vi "Wärmepumpe.WriteZustandsgrössen.vi"(0 "Wärmepumpe in":refnum<data-value>, 1 "Vorlauftemperatur \nHeizkreislauf [°C] WPM":dbl, 2 "Vorlauftemperatur \nSolekreislauf [°C] WPM":dbl, 3 "Verdichter 1":bool, 4 "Verdichter 2":bool, 5 "Error in":errorcluster) -> (19 "Error out":errorcluster)   [LabVIEW 2016, in "Wärmepumpe.lvclass"]
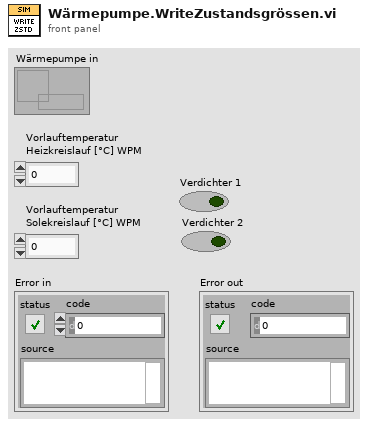
[diagram p1: front panel]
types:
  T1 = typedef "Wärmepumpe.lvclass/Wärmepumpe.Zustandsgrössen.ctl" = cluster{"Vorlauftemperatur Heizkreislauf[°C]":dbl, "Vorlauftemperatur Solekreislauf[°C]":dbl, "Heizleistung [W]":dbl, "Kälteleistung [W]":dbl, "Verdichter 1":bool, "Verdichter 2":bool}
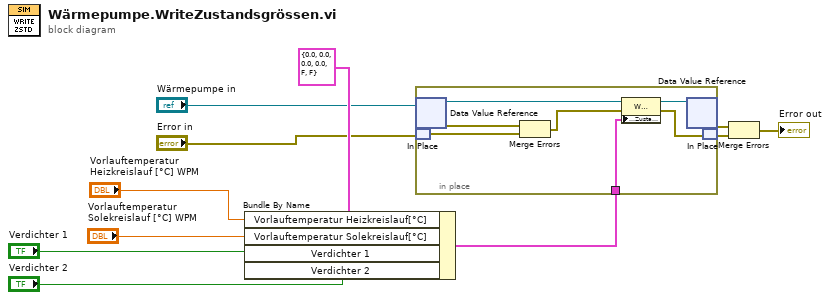
[diagram p0: block diagram]
diagram:
  n1 = Bundle By Name(cluster=T1 {"Vorlauftemperatur Heizkreislauf[°C]"=0.0, "Vorlauftemperatur Solekreislauf[°C]"=0.0, "Heizleistung [W]"=0.0, "Kälteleistung [W]"=0.0, "Verdichter 1"=FALSE, "Verdichter 2"=FALSE} ("Wärmepumpe.Zustandsgrössen"), "Vorlauftemperatur Heizkreislauf[°C]"="Vorlauftemperatur \nHeizkreislauf [°C] WPM", "Vorlauftemperatur Solekreislauf[°C]"="Vorlauftemperatur \nSolekreislauf [°C] WPM", "Verdichter 1"="Verdichter 1", "Verdichter 2"="Verdichter 2") -> (w6:T1)
  n2 = in-place {
    in-place-border: w6 -> [w12]
    n3 = in-place-dvr #1("Wärmepumpe in") -> (w18:refnum<class "Wärmepumpe.lvclass">, w15:errorcluster)
    n4 = in-place-match #2("Error in") -> (w14:errorcluster)
    n5 = Merge Errors(w15, w14) -> (w16:errorcluster)
    n6 = property class="Wärmepumpe.lvclass"(reference=w18, error in=w16, "Accessors:Wärmepumpe.Zustandsgrössen"=w12) -> (reference out=w17:refnum<class "Wärmepumpe.lvclass">, error out=w13:errorcluster)
    n7 = in-place-dvr #1(w17) -> (w10:errorcluster)  [unwired: 1 out]
    n8 = in-place-match #2(w13) -> (w9:errorcluster)
  }
  n9 = Merge Errors(w10, w9) -> (→"Error out":errorcluster)
